vi "Editor_vinculo_instrumento_PDF.vi"() -> ()   [LabVIEW 2019]
uses:
  <vilib>/Utility/config.llb/Config Data RefNum.ctl
  <vilib>/Utility/config.llb/Write Key (String).vi
  <vilib>/Utility/config.llb/Read Key (String).vi
  <vilib>/Utility/config.llb/NI_LVConfig.lvlib
panel:
  in  "Search Button":bool
  in  "barra_de_pesquisa":string
  out "path certificados":path
  in  "Abrir outros":bool
  in  "Cancel Button":bool
  in  "Save Button":bool
  in  "Array":cluster{"TAG":string, "path":path}[](array[cluster])
  in  "Stop Button":bool
  out "array nao moficado":cluster{"TAG":string, "path":path}[](array[cluster])
  out "error out":errorcluster
  out "refnum out":T1
  out "Section Names":string[](array[string])
  # "Digite no campo de busca a TAG desejada:"
  # "EDITE O CAMINHO PATH DO \nCERTIFICADO DE CALIBRA敲O\nCOM SUA RESPECTIVA TAG"
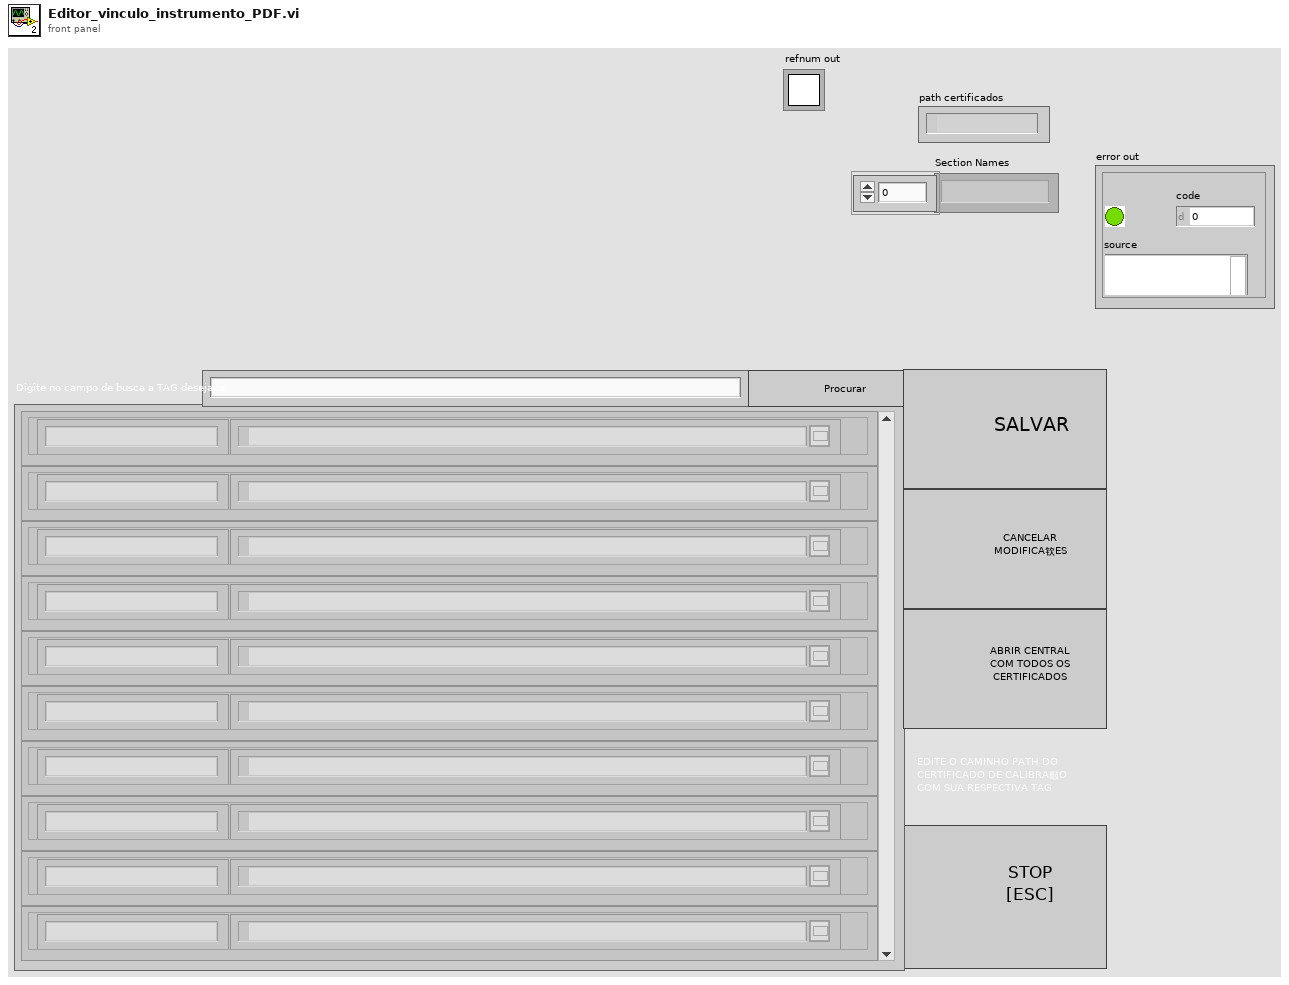
[diagram p1: front panel]
types:
  T1 = typedef "NI_LVConfig.lvlib/Config Data RefNum.ctl" = refnum<k1>
  T2 = enum8{"Enabled", "Disabled", "Disabled and Grayed Out"}
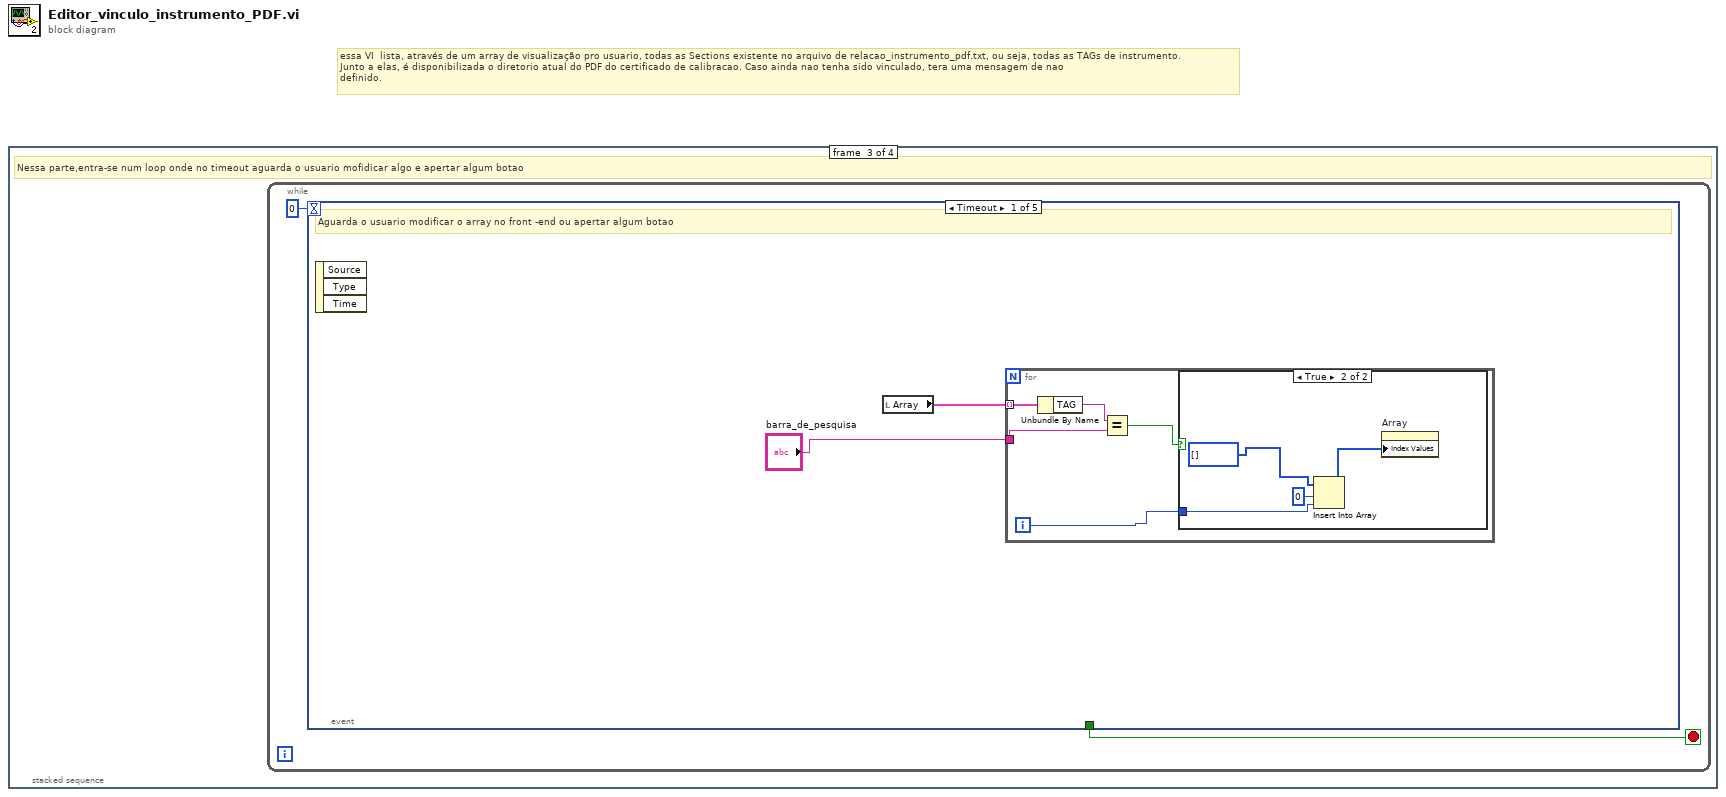
[diagram p0: block diagram]
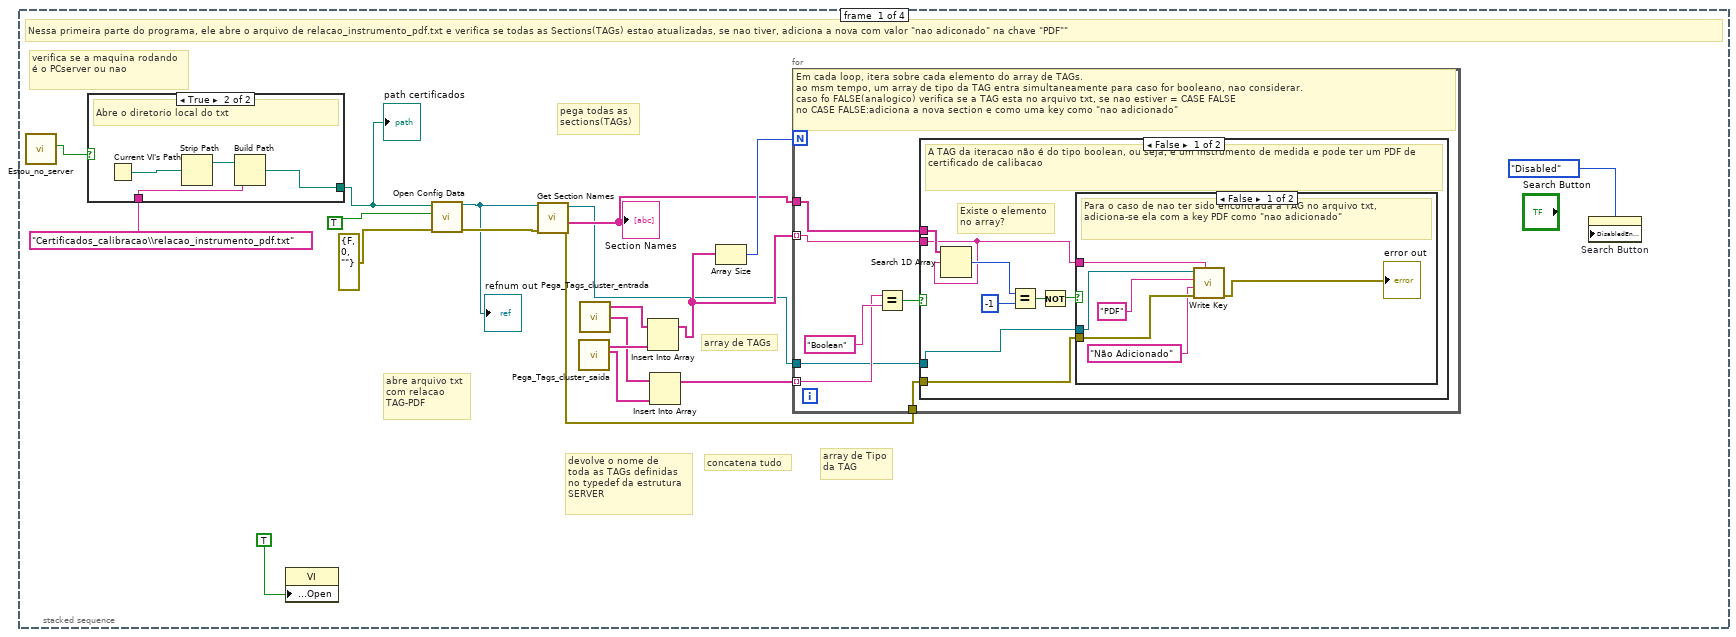
[diagram p2: hidden frame]
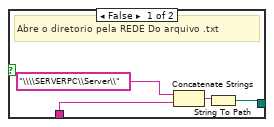
[diagram p3: hidden frame]
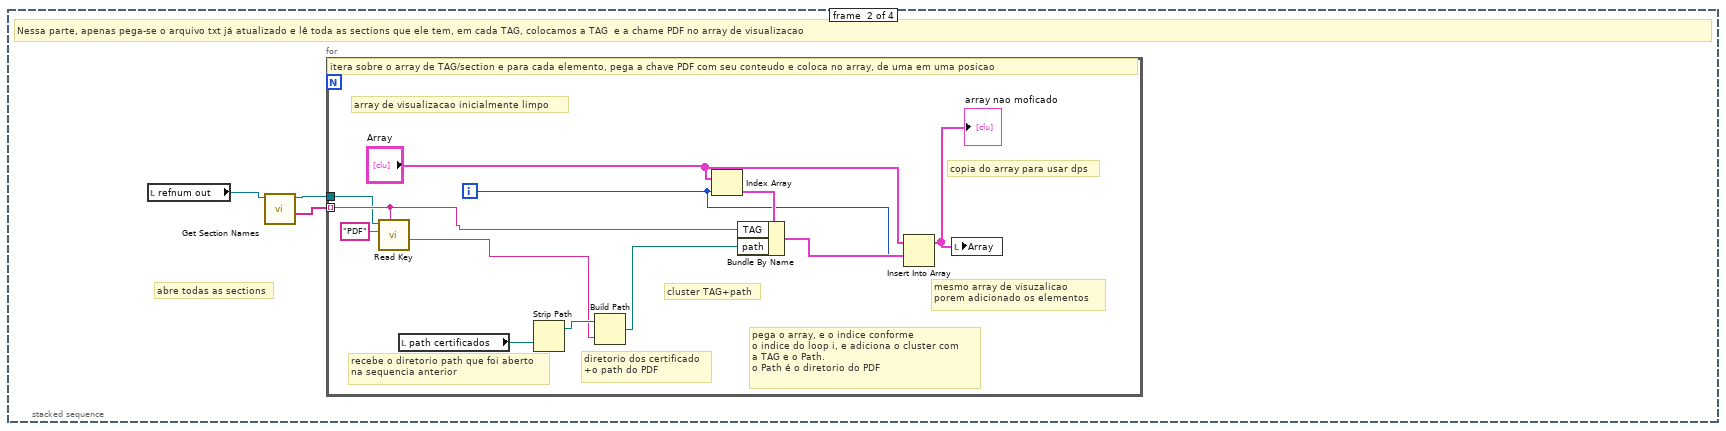
[diagram p6: hidden frame]
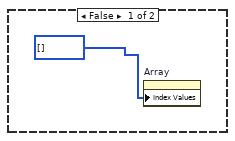
[diagram p7: hidden frame]
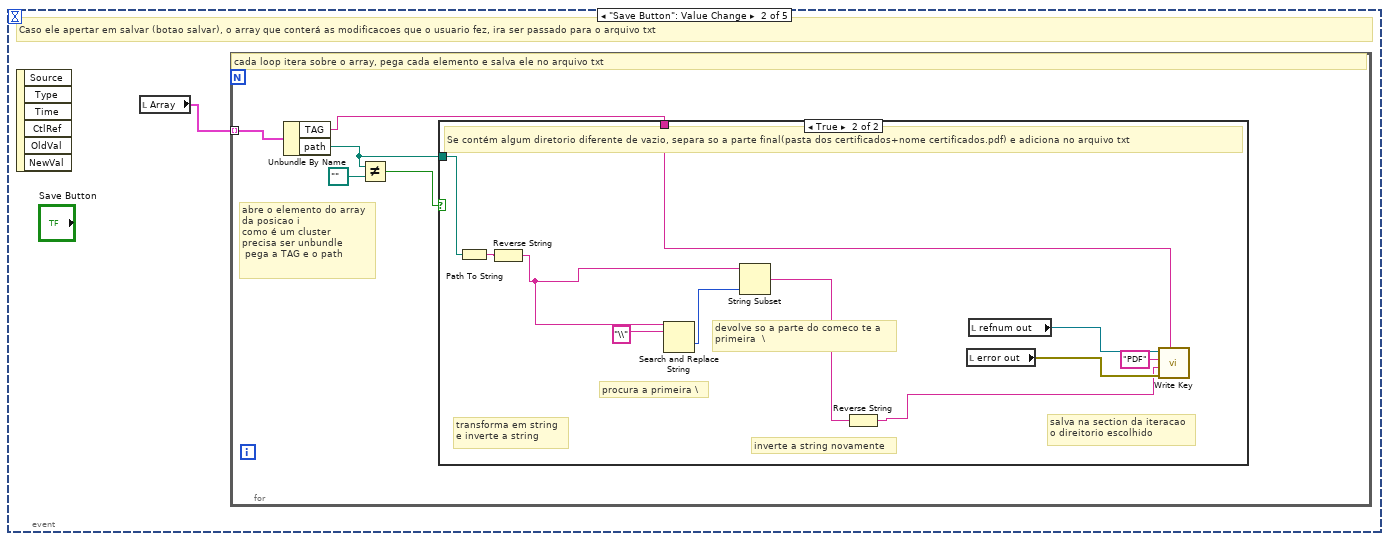
[diagram p8: hidden frame]
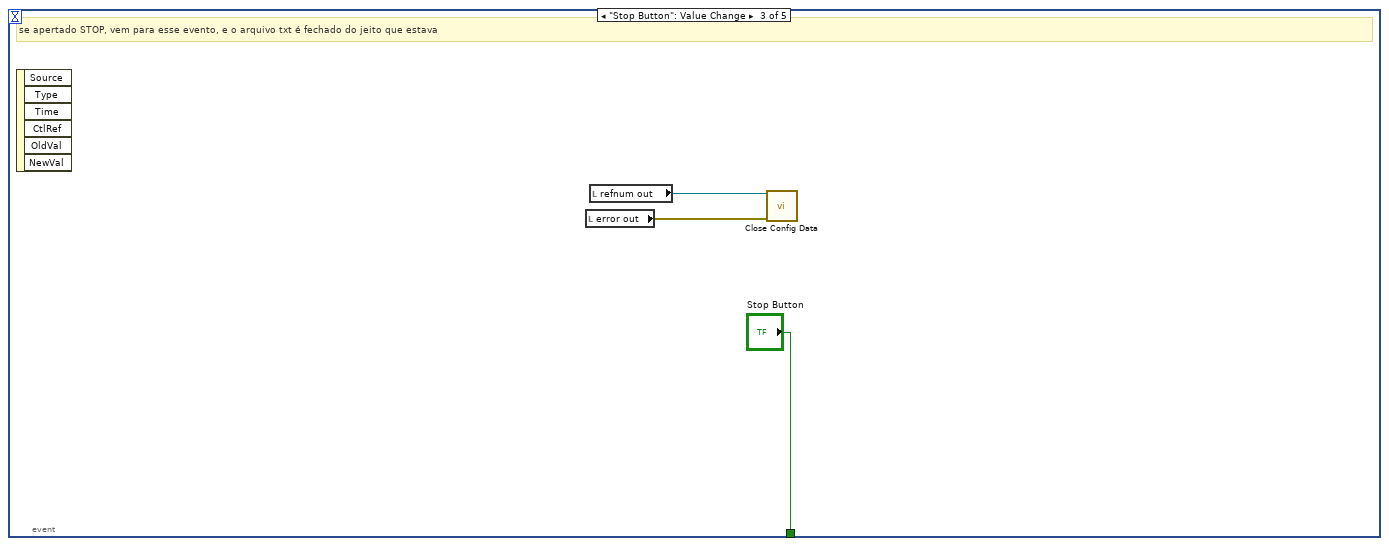
[diagram p10: hidden frame]
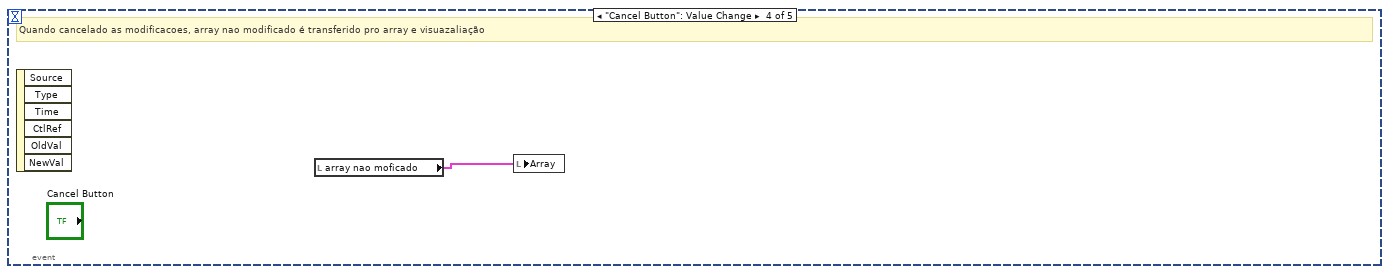
[diagram p11: hidden frame]
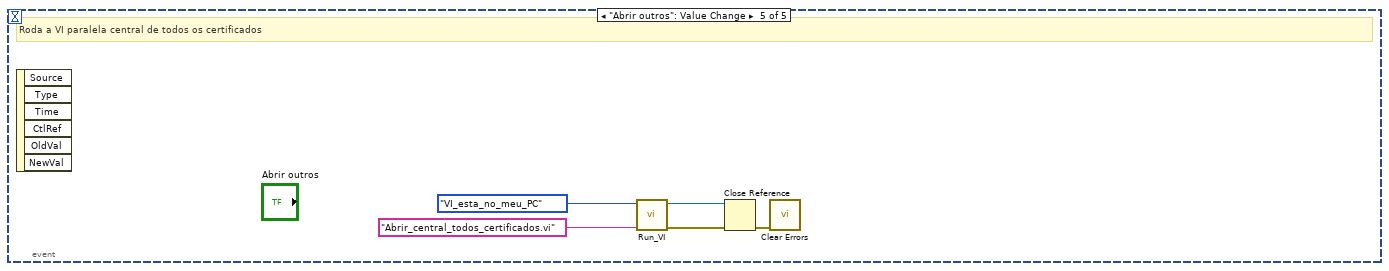
[diagram p12: hidden frame]
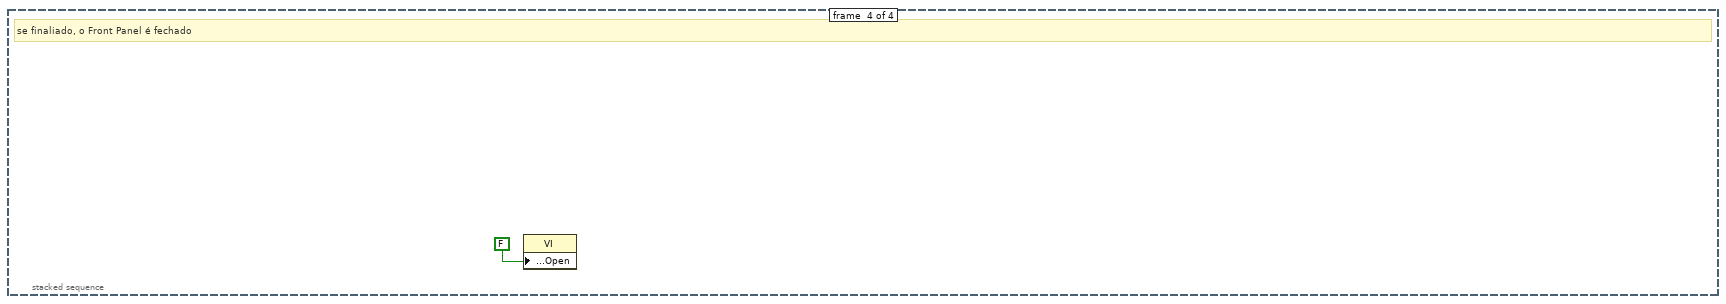
[diagram p13: hidden frame]
diagram:
  # "essa VI  lista, através de um array de visualização pro usuario, todas as Sections existente no arquivo de relacao_instrumento_pdf.txt, ou seja, todas as TAGs de instrumento.\nJunto a elas, é disponibilizada o diretorio atual do PDF do certificado de calibracao. Caso ainda nao tenha sido vinculado, tera uma mensagem de nao \ndefinido."
  n1 = stacked-sequence {
    frame #0 {
      # "array de Tipo\nda TAG"
      # "array de TAGs"
      # "concatena tudo"
      # "devolve o nome de\ntoda as TAGs definidas\nno typedef da estrutura\nSERVER"
      # "pega todas as\nsections(TAGs)"
      # "abre arquivo txt\ncom relacao\nTAG-PDF"
      # "verifica se a maquina rodando é o PCserver ou nao"
      # "Nessa primeira parte do programa, ele abre o arquivo de relacao_instrumento_pdf.txt e verifica se todas as Sections(TAGs) estao atualizadas, se nao tiver, adiciona a nova com valor \"nao adiconado\" na chave \"PDF\"\""
      n2 = call "Estou_no_server.vi"() -> ("Estou no serve?"=w3:bool)  [unwired: 11 in]
      n3 = case shown="True" w3 {
        tunnel: [w21 w26] -> w2
        tunnel: "Certificados_calibracao\\relacao_instrumento_pdf.txt" ("name or relative path") -> [w22 w25]
        frame False {
          # "Abre o diretorio pela REDE Do arquivo .txt"
          n4 = Concatenate Strings("\\\\SERVERPC\\Server\\", w22) -> (w20:string)
          n5 = String To Path(string=w20) -> (path=w21:path)
        }
        frame True {
          # "Abre o diretorio local do txt"
          n6 = Current VI's Path() -> (path=w24:path)
          n7 = Strip Path(path=w24) -> (stripped path=w27:path)  [unwired: 1 out]
          n8 = Build Path(base path=w27, name or relative path=w25) -> (appended path=w26:path)
        }
      }
      "path certificados" <- w2
      n9 = property class="VI"("Front Panel.Open"=TRUE ("Front Panel Window:Open")) -> ()  [unwired: 2 in, 2 out]
      n10 = call <vilib>:"Open Config Data.vi"("error in (no error)"=errorcluster {"status"=FALSE, "code"=0, "source"=""}, "create file if necessary (T)"=TRUE, "configuration file path"=w2) -> ("error out"=w16:errorcluster, "refnum"=w15:T1)  [unwired: 6 in, 1 out]
      "refnum out" <- w15
      n11 = call <vilib>:"Get Section Names.vi"("error in (no error)"=w16, "refnum"=w15) -> ("error out"=w5:errorcluster, "section names"=w11:string[], "refnum out"=w6:T1)  [unwired: 7 in]
      "Section Names" <- w11
      n12 = call "Pega_Tags_cluster_saida.vi"() -> ("TipoTag"=w8:string[], "Array Tags"=w13:string[])  [unwired: 10 in]
      n13 = call "Pega_Tags_cluster_entrada.vi"() -> ("TipoVariavel"=w9:string[], "Array Tags"=w14:string[])  [unwired: 4 in]
      n14 = Insert Into Array(array=w14, new element=w13) -> (w10:string[])  [unwired: 1 in]
      n15 = Insert Into Array(array=w9, new element=w8) -> (w7:string[])  [unwired: 1 in]
      n16 = Array Size(array=w10) -> (size(s)=w12:i32)
      n17 = for {
        N: w12 -> [_]
        tunnel: w10 -> [w31] mode=indexing
        tunnel: w11 -> [w30]
        tunnel: w7 -> [w33] mode=indexing
        tunnel: w6 -> [w29]
        tunnel: w5 -> [w28]
        # "Em cada loop, itera sobre cada elemento do array de TAGs.\nao msm tempo, um array de tipo da TAG entra simultaneamente para caso for booleano, nao considerar.\ncaso fo FALSE(analogico) verifica se a TAG esta no arquivo txt, se nao estiver = CASE FALSE\nno CASE FALSE:adiciona a nova section e como uma key como \"nao adicionado\""
        n18 = Equal?(x=w33, y="Boolean") -> (x = y?=w32:bool)
        n19 = case shown="False" w32 {
          tunnel: w31 -> [w37 _]
          tunnel: w30 -> [w40 _]
          tunnel: w29 -> [w36 _]
          tunnel: w28 -> [w35 _]
          frame False {
            # "Existe o elemento\nno array?"
            # "A TAG da iteracao não é do tipo boolean, ou seja, é um instrumento de medida e pode ter um PDF de certificado de calibacao"
            n20 = Search 1D Array(1D array=w40, element=w37) -> (index of element=w39:i32)  [unwired: 1 in]
            n21 = Equal?(x=w39, y=-1) -> (x = y?=w42:bool)
            n22 = Not(x=w42) -> (.not. x?=w38:bool)
            n23 = case shown="False" w38 {
              tunnel: w37 -> [w48 _]
              tunnel: w36 -> [w46 _]
              tunnel: w35 -> [w45 _]
              frame False {
                # "Para o caso de nao ter sido encontrada a TAG no arquivo txt,\nadiciona-se ela com a key PDF como \"nao adicionado\""
                n24 = call-poly <vilib>:"Write Key.vi"("section"=w48, "error in (no error)"=w45, "value"="Não Adicionado", "key"="PDF", "refnum"=w46) -> ("error out"=→"error out":errorcluster)  [unwired: 4 in, 2 out]
              }
              frame True {
              }
            }
          }
          frame True {
            # "a TAG analisada é uma booleana"
          }
        }
      }
      n25 = property on="Search Button" class="Bool"("DisabledEnum"=T2."Disabled" ("Disabled")) -> ()  [unwired: 2 in, 2 out]
    }
    frame #1 {
      # "abre todas as sections"
      # "Nessa parte, apenas pega-se o arquivo txt já atualizado e lê toda as sections que ele tem, em cada TAG, colocamos a TAG  e a chame PDF no array de visualizacao"
      n26 = local read "refnum out"() -> (w51:T1)
      n27 = call <vilib>:"Get Section Names.vi"("refnum"=w51) -> ("section names"=w50:string[], "refnum out"=w49:T1)  [unwired: 8 in, 1 out]
      n28 = for {
        tunnel: w50 -> [w58] mode=indexing
        tunnel: w49 -> [w56]
        i -> [w61]
        # "copia do array para usar dps"
        # "mesmo array de visuzalicao\nporem adicionado os elementos"
        # "array de visualizacao inicialmente limpo"
        # "diretorio dos certificado\n+o path do PDF"
        # "recebe o diretorio path que foi aberto\nna sequencia anterior"
        # "cluster TAG+path"
        # "pega o array, e o indice conforme\no indice do loop i, e adiciona o cluster com\na TAG e o Path.\no Path é o diretorio do PDF"
        # "itera sobre o array de TAG/section e para cada elemento, pega a chave PDF com seu conteudo e coloca no array, de uma em uma posicao"
        n29 = call-poly <vilib>:"Read Key.vi"("section"=w58, "key"="PDF", "refnum"=w56) -> ("value"=w52:string)  [unwired: 5 in, 3 out]
        n30 = local read "path certificados"() -> (w54:path)
        n31 = Strip Path(path=w54) -> (stripped path=w53:path)  [unwired: 1 out]
        n32 = Build Path(base path=w53, name or relative path=w52) -> (appended path=w55:path)
        n33 = Index Array(array="Array", index=w61) -> (element=w63:cluster{"TAG":string, "path":path})
        n34 = Bundle By Name(cluster=w63, "TAG"=w58, "path"=w55) -> (w62:cluster{"TAG":string, "path":path})
        n35 = Insert Into Array(array="Array", index=w61, new element=w62) -> (w59:cluster{"TAG":string, "path":path}[])
        "array nao moficado" <- w59
        n36 = local write "Array"(w59) -> ()
      }
    }
    frame #2 {
      # "Nessa parte,entra-se num loop onde no timeout aguarda o usuario mofidicar algo e apertar algum botao"
      n37 = while {
        stop <- w65 stop-if-true
        n38 = event shown="[0] Timeout" {
          selector: _ -> [_ _ _ _ _]
          dyn-events: _ -> [_ _ _ _ _]
          timeout: 0 -> [_ _ _ _ _]
          tunnel: [_ _ "Stop Button" _ _] -> w65
          event Timeout {
            # "Aguarda o usuario modificar o array no front -end ou apertar algum botao"
            n39 = event-data() -> ()  [unwired: 1 in, 3 out]
            n40 = local read "Array"() -> (w67:cluster{"TAG":string, "path":path}[])
            n41 = for {
              tunnel: w67 -> [w72] mode=indexing
              tunnel: "barra_de_pesquisa" -> [w70]
              i -> [w69]
              n42 = Unbundle By Name(w72) -> ("TAG"=w71:string)
              n43 = Equal?(x=w71, y=w70) -> (x = y?=w68:bool)
              n44 = case shown="True" w68 {
                tunnel: w69 -> [_ w76]
                frame False {
                  n45 = property on="Array" class="Arr (strict)"("Index Values"=u32[] []) -> ()  [unwired: 2 in, 2 out]
                }
                frame True {
                  n46 = Insert Into Array(array=u32[] [] ("Index Values"), index=0, new element=w76) -> (w74:u32[])
                  n47 = property on="Array" class="Arr (strict)"("Index Values"=w74) -> ()  [unwired: 2 in, 2 out]
                }
              }
            }
          }
          event "Save Button": Value Change {
            # "Caso ele apertar em salvar (botao salvar), o array que conterá as modificacoes que o usuario fez, ira ser passado para o arquivo txt"
            n48 = event-data() -> ()  [unwired: 1 in, 6 out]
            n49 = local read "Array"() -> (w78:cluster{"TAG":string, "path":path}[])
            n50 = for {
              tunnel: w78 -> [w83] mode=indexing
              # "abre o elemento do array\nda posicao i\ncomo é um cluster\nprecisa ser unbundle\n pega a TAG e o path"
              # "cada loop itera sobre o array, pega cada elemento e salva ele no arquivo txt"
              n51 = Unbundle By Name(w83) -> ("TAG"=w80:string, "path"=w79:path)
              n52 = Not Equal?(x=w79, y=path "") -> (x != y?=w81:bool)
              n53 = case shown="True" w81 {
                tunnel: w80 -> [_ w92]
                tunnel: w79 -> [_ w86]
                frame False {
                  # "se o path é igual a Vazio, nao faz nada"
                }
                frame True {
                  # "salva na section da iteracao\no direitorio escolhido"
                  # "inverte a string novamente"
                  # "devolve so a parte do comeco te a\nprimeira  \\"
                  # "procura a primeira \\"
                  # "transforma em string\ne inverte a string"
                  # "Se contém algum diretorio diferente de vazio, separa so a parte final(pasta dos certificados+nome certificados.pdf) e adiciona no arquivo txt"
                  n54 = Path To String(path=w86) -> (string=w85:string)
                  n55 = Reverse String(1:w85) -> (0:w88:string)
                  n56 = Search and Replace String(input string=w88, search string="\\") -> (offset past replacement=w89:i32)  [unwired: 6 in, 3 out]
                  n57 = String Subset(string=w88, length (rest)=w89) -> (substring=w87:string)  [unwired: 1 in]
                  n58 = Reverse String(1:w87) -> (0:w84:string)
                  n59 = local read "error out"() -> (w93:errorcluster)
                  n60 = local read "refnum out"() -> (w94:T1)
                  n61 = call-poly <vilib>:"Write Key.vi"("section"=w92, "error in (no error)"=w93, "value"=w84, "key"="PDF", "refnum"=w94) -> ()  [unwired: 4 in, 3 out]
                }
              }
            }
          }
          event "Stop Button": Value Change {
            # "se apertado STOP, vem para esse evento, e o arquivo txt é fechado do jeito que estava"
            n62 = event-data() -> ()  [unwired: 1 in, 6 out]
            n63 = local read "error out"() -> (w95:errorcluster)
            n64 = local read "refnum out"() -> (w96:T1)
            n65 = call <vilib>:"Close Config Data.vi"("error in (no error)"=w95, "refnum"=w96) -> ()  [unwired: 8 in, 2 out]
          }
          event "Cancel Button": Value Change {
            # "Quando cancelado as modificacoes, array nao modificado é transferido pro array e visuazaliação"
            n66 = event-data() -> ()  [unwired: 1 in, 6 out]
            n67 = local read "array nao moficado"() -> (w98:cluster{"TAG":string, "path":path}[])
            n68 = local write "Array"(w98) -> ()
          }
          event "Abrir outros": Value Change {
            # "Roda a VI paralela central de todos os certificados"
            n69 = event-data() -> ()  [unwired: 1 in, 6 out]
            n70 = call "Run_VI.vi"("Nome.vi"="Abrir_central_todos_certificados.vi", "Origem_VI"=enum16{"VI_esta_no_meu_PC", "VI_esta_na_rede"}."VI_esta_no_meu_PC") -> ("error out"=w102:errorcluster, "reference out"=w103:refnum<vi>)  [unwired: 8 in]
            n71 = Close Reference(reference=w103, error in (no error)=w102) -> (error out=w101:errorcluster)
            n72 = call <vilib>:"Clear Errors.vi"("error in (no error)"=w101) -> ()  [unwired: 5 in, 2 out]
          }
        }
      }
    }
    frame #3 {
      # "se finaliado, o Front Panel é fechado"
      n73 = property class="VI"("Front Panel.Open"=FALSE ("Front Panel Window:Open")) -> ()  [unwired: 2 in, 2 out]
    }
  }
